vi "Configure Relative Offset.vi"(5 "Enable Relative (F: Disable)":bool, 6 "Method (0: Parts)":i32(ring) items=["Parts", "Result"], 7 "Offset (0)":dbl, 8 "error in (no error)":errorcluster, 9 "Channel List (\"\")":string, 10 "Function (0: Voltage DC)":i32(ring) items=[" Voltage DC", "Voltage AC", "Current DC", "Current AC", "Resistance", "4-wire Resistance", "Diode", "Capacitance", "Temperature", "Continuity", "Frequency", "Period", "Voltage Ratio", "Digitize Voltage", "Digitize Current"], 11 "VISA resource name":refnum<visa-resource-name>) -> (0 "error out":errorcluster, 3 "VISA resource name out":refnum<visa-resource-name>)   [LabVIEW 2020, in "Keithley DMM6500 DAQ6500 Series.lvlib"]
doc: "Configures the application of a relative offset value to the measurement."
uses:
  <instrlib>/Keithley DMM6500 DAQ6500 Series/Keithley DMM6500 DAQ6500 Series.lvlib
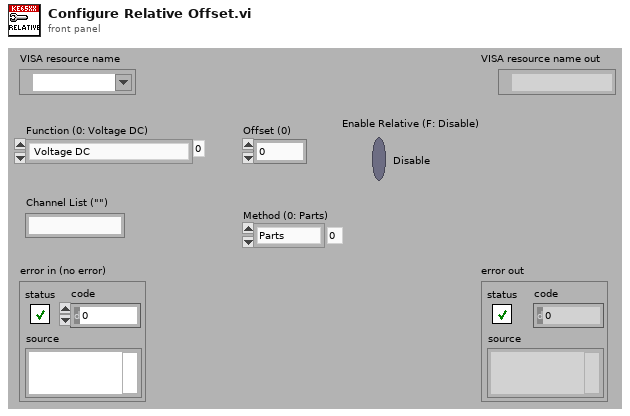
[diagram p1: front panel]
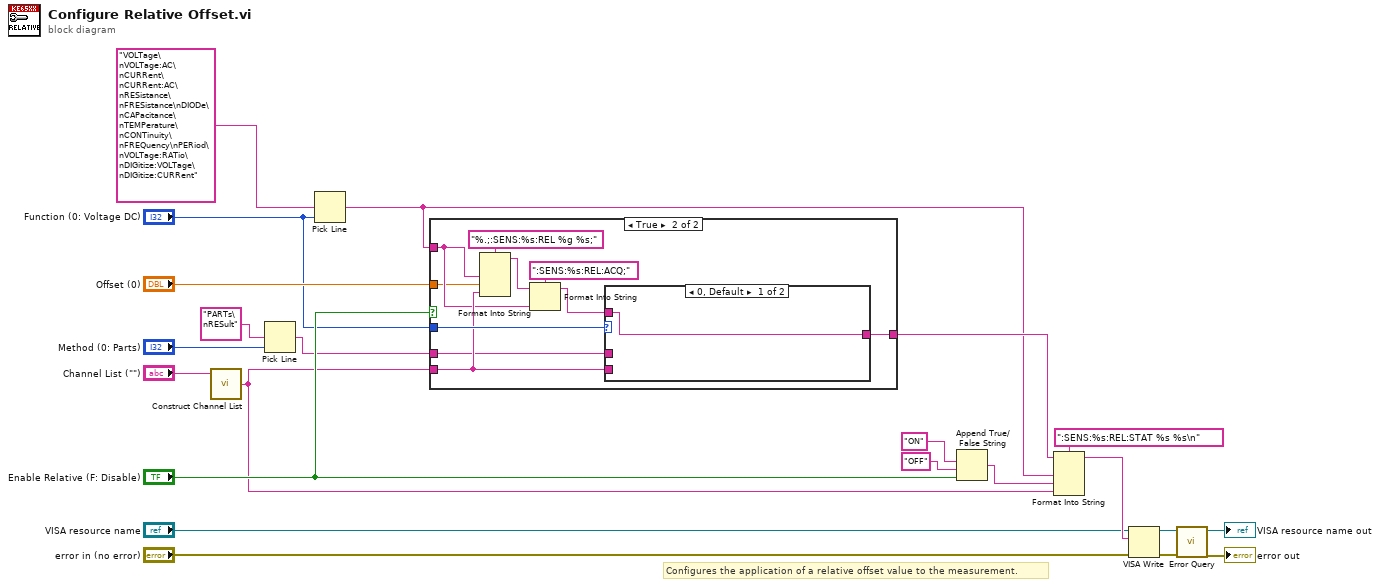
[diagram p0: block diagram]
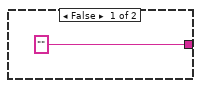
[diagram p2: hidden frame]
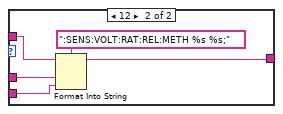
[diagram p3: hidden frame]
diagram:
  # "Configures the application of a relative offset value to the measurement."
  n1 = call <instrlib>:"Construct Channel List.vi"("Channel List"="Channel List (\"\")") -> ("Channel List String"=w7:string)  [unwired: 2 in]
  n2 = Pick Line(multi-line string="PARTs\nRESult", line index="Method (0: Parts)") -> (output string=w2:string)  [unwired: 1 in]
  n3 = Pick Line(multi-line string="VOLTage\nVOLTage:AC\nCURRent\nCURRent:AC\nRESistance\nFRESistance\nDIODe\nCAPacitance\nTEMPerature\nCONTinuity\nFREQuency\nPERiod\nVOLTage:RATio\nDIGitize:VOLTage\nDIGitize:CURRent", line index="Function (0: Voltage DC)") -> (output string=w6:string)  [unwired: 1 in]
  n4 = case shown="True" "Enable Relative (F: Disable)" {
    tunnel: ["" w29] -> w20
    tunnel: "Function (0: Voltage DC)" -> [_ w28]
    tunnel: w7 -> [_ w27]
    tunnel: w6 -> [_ w26]
    tunnel: "Offset (0)" -> [_ w25]
    tunnel: w2 -> [_ w24]
    frame False {
    }
    frame True {
      n5 = Format Into String(format string="%.;:SENS:%s:REL %g %s;", w26, w25, w27) -> (resulting string=w32:string)  [unwired: 2 in, 1 out]
      n6 = Format Into String(format string=":SENS:%s:REL:ACQ;", initial string=w32, w26) -> (resulting string=w30:string)  [unwired: 1 in, 1 out]
      n7 = case shown="0, Default" w28 {
        tunnel: w30 -> [w34 w35]
        tunnel: [w34 w38] -> w29
        tunnel: w27 -> [_ w37]
        tunnel: w24 -> [_ w36]
        frame 0, Default {
        }
        frame 12 {
          n8 = Format Into String(format string=":SENS:VOLT:RAT:REL:METH %s %s;", initial string=w35, w36, w37) -> (resulting string=w38:string)  [unwired: 1 in, 1 out]
        }
      }
    }
  }
  n9 = Append True/False String(1:"Enable Relative (F: Disable)", 2:"OFF", 3:"ON") -> (0:w18:string)  [unwired: 1 in]
  n10 = Format Into String(format string=":SENS:%s:REL:STAT %s %s\n", initial string=w20, w6, w18, w7) -> (resulting string=w17:string)  [unwired: 1 in, 1 out]
  n11 = VISA Write(VISA resource name="VISA resource name", write buffer=w17, error in (no error)="error in (no error)") -> (VISA resource name out=w14:refnum<visa-resource-name>, error out=w13:errorcluster)  [unwired: 1 out]
  n12 = call <instrlib>:"Error Query.vi"("error in (no error)"=w13, "VISA resource name"=w14) -> ("error out"=→"error out":errorcluster, "VISA resource name out"=→"VISA resource name out":refnum<visa-resource-name>)  [unwired: 6 in, 2 out]
